vi "Get S34CON wrapper.vi"(8 "error in (no error)":errorcluster caption="错误输入（无错误）", 10 "dwCanNodeId":u32, 11 "dwDevIndex":u32) -> (0 "error out":errorcluster caption="错误输出", 1 "S34CON":T1, 3 "function return":u32)   [LabVIEW 2016, in "UISimCanFunc_wrapper.lvlib"]
doc: "_declspec (dllexport) DWORD GetS34CON_wrapper(DWORD dwDevIndex, DWORD dwCanNodeId, P_S34CON pS34Con);"
uses:
  <userlib>/UISimCanFunc_wrapper/UISimCanFunc_wrapper.lvlib
  <userlib>/UISimCanFunc_wrapper/ctl/S34CON.ctl
  <userlib>/UISimCanFunc_wrapper/UISimCanFunc_wrapper.dll
panel:
  in  "pS34Con":T2
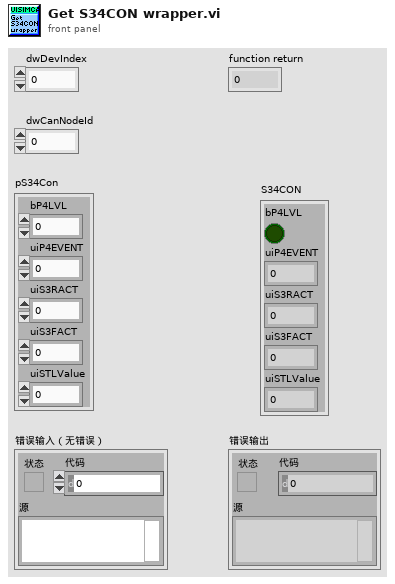
[diagram p1: front panel]
types:
  T1 = typedef "UISimCanFunc_wrapper.lvlib/S34CON.ctl" = cluster{"bP4LVL":bool, "uiP4EVENT":u32, "uiS3RACT":u32, "uiS3FACT":u32, "uiSTLValue":u32}
  T2 = cluster{"bP4LVL":i32, "uiP4EVENT":u32, "uiS3RACT":u32, "uiS3FACT":u32, "uiSTLValue":u32}
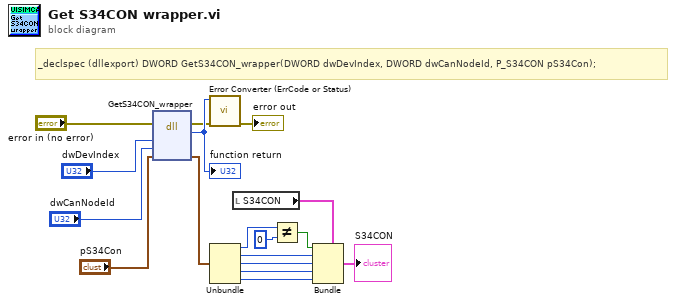
[diagram p0: block diagram]
diagram:
  # "_declspec (dllexport) DWORD GetS34CON_wrapper(DWORD dwDevIndex, DWORD dwCanNodeId, P_S34CON pS34Con);"
  n1 = dll-call lib="C:/Program Files (x86)/National Instruments/LabVIEW 2016/user.lib/UISimCanFunc_wrapper/UISimCanFunc_wrapper.*" fn="GetS34CON_wrapper"(error in="error in (no error)", "dwDevIndex"="dwDevIndex", "dwCanNodeId"="dwCanNodeId", "pS34Con"="pS34Con") -> (error out=w12:errorcluster, w17:u32, "pS34Con"=w8:T2)  [unwired: 4 in, 1 out]
  "function return" <- w17
  n2 = call <userlib>:"Error Converter (ErrCode or Status).vi"("error in (no error)"=w12, "error code"=w17) -> ("error out"=→"error out":errorcluster)  [unwired: 9 in]
  n3 = Unbundle(w8) -> ("bP4LVL"=w6:i32, "uiP4EVENT"=w4:u32, "uiS3RACT"=w3:u32, "uiS3FACT"=w2:u32, "uiSTLValue"=w1:u32)
  n4 = local read "S34CON"() -> (w10:T1)
  n5 = Not Equal?(x=w6, y=0) -> (x != y?=w5:bool)
  n6 = Bundle(cluster=w10, "bP4LVL"=w5, "uiP4EVENT"=w4, "uiS3RACT"=w3, "uiS3FACT"=w2, "uiSTLValue"=w1) -> (→"S34CON":T1)
